vi "PolyTec_Control_Panel.vi"(11 "Settings in":T3={"Name of test"="ScratchPad", "Date"=timestamp(3622387832 s since 1904-01-01), "Location"="Home", "Template"="ScratchPad", "Soundcard"="Babyface Pro (71982712)", "resolution"=32, "Sampling rate"=48000, "Ch1 Gain "=15.0, "Ch2 Gain"=20.0, "Sample time (s)"=0.3, "Pre-trigger (s)"=0.001, "Hammer Threshold"=0.05, "Positions"=1, "Taps/Position"=5, "Set Names"="H", "Freq resolution"=1.0, "Hammer cutoff"=0.03, "Mic cutoff"=0.1, "Double bounce "=0.01, "Hammer Cal"=1.0, "dB Offset"=0.0, "Accel Cal"=1.0, "Vibrometer Cal"=20.0, "Mic Cal"=49.38, "Output"=2, "Voltage Cal"=13.4, "Vibrometer Port"="ASRL27::INSTR", "Range"=4, "High Pass"=2, "Bandwidth"=4, "X Range"=[{"Minimum"=200.0, "Maximum"=10000.0, "Increment"=10.0, "Minor Increment"=100.0, "Start"=200.0}, {"Minimum"=0.0, "Maximum"=0.05, "Increment"=0.025, "Minor Increment"=0.0025, "Start"=0.0}, {"Minimum"=0.0, "Maximum"=0.3, "Increment"=0.1, "Minor Increment"=0.01, "Start"=0.0}, {"Minimum"=200.0, "Maximum"=10000.0, "Increment"=10.0, "Minor Increment"=100.0, "Start"=1000.0}], "Y Range"=[{"Minimum"=-25.0, "Maximum"=0.0, "Increment"=5.0, "Minor Increment"=1.0, "Start"=-25.0}, {"Minimum"=-0.01, "Maximum"=0.1, "Increment"=0.02, "Minor Increment"=0.005, "Start"=0.0}, {"Minimum"=-0.1, "Maximum"=0.1, "Increment"=0.05, "Minor Increment"=0.01, "Start"=-0.1}, {"Minimum"=-61.0, "Maximum"=-21.0, "Increment"=2.0, "Minor Increment"=0.5, "Start"=-60.0}], "dB Spread"=40.0, "Trigger"=0, "Ch_1"=2, "Ch_2"=1, "flip?"=FALSE, "60Hz"=FALSE, "Time offset"=0.0, "Piezo Cal"=1.0, "Default Notes"=""} {"Ch_2" min=1 step=1; "Ch_1" min=1 max=100 step=1; "Trigger" items=["Hammer (force)", "Self-tap", "Spacebar"]; "Bandwidth" items=["1 kHz"=1, "5 kHz"=5, "10 kHz"=10, "25 kHz"=25, "50 kHz"=50, "100 kHz"=100]; "High Pass" items=["Off", "13 Hz", "104 Hz"]; "Range" items=["10 mm/s"=1, "20 mm/s"=2, "50 mm/s"=5, "100 mm/s"=10, "200 mm/s"=20, "500 mm/s"=50, "1 m/s"=100, "2 m/s"=200]; "Output" items=["Accelerometer", "Speed (from acceleration)", "Microphone", "Vibrometer", "Piezo"]; "Voltage Cal" format="%#_13g"; "Ch2 Gain" format="%#_13g"; "Ch1 Gain" format="%#_13g"; "Double bounce" min=0.0; "Mic cutoff" min=0.0 format="%#_4g"; "Hammer cutoff" min=0.0 format="%#_4g"; "Freq resolution" min=0.0; "Pre-trigger (s)" format="%#_13g"; "Date" format="%<%H:%M\n%d/%m/%y>T"; "resolution" items=["16 bit"=16, "24 bit"=24, "32 bit"=32]; "Sampling rate" items=["22050 samp/s"=22050, "44100 samp/s"=44100, "48000 samp/s"=48000]}) -> (1 "Success?":bool, 2 "Updated Settings":T4, 3 "Settings Out":T3={"Name of test"="ScratchPad", "Date"=timestamp(3622387832 s since 1904-01-01), "Location"="Home", "Template"="ScratchPad", "Soundcard"="Babyface Pro (71982712)", "resolution"=32, "Sampling rate"=48000, "Ch1 Gain "=15.0, "Ch2 Gain"=20.0, "Sample time (s)"=0.3, "Pre-trigger (s)"=0.001, "Hammer Threshold"=0.05, "Positions"=1, "Taps/Position"=5, "Set Names"="H", "Freq resolution"=1.0, "Hammer cutoff"=0.03, "Mic cutoff"=0.1, "Double bounce "=0.01, "Hammer Cal"=1.0, "dB Offset"=0.0, "Accel Cal"=1.0, "Vibrometer Cal"=20.0, "Mic Cal"=49.38, "Output"=2, "Voltage Cal"=13.4, "Vibrometer Port"="ASRL27::INSTR", "Range"=4, "High Pass"=2, "Bandwidth"=4, "X Range"=[{"Minimum"=200.0, "Maximum"=10000.0, "Increment"=10.0, "Minor Increment"=100.0, "Start"=200.0}, {"Minimum"=0.0, "Maximum"=0.05, "Increment"=0.025, "Minor Increment"=0.0025, "Start"=0.0}, {"Minimum"=0.0, "Maximum"=0.3, "Increment"=0.1, "Minor Increment"=0.01, "Start"=0.0}, {"Minimum"=200.0, "Maximum"=10000.0, "Increment"=10.0, "Minor Increment"=100.0, "Start"=1000.0}], "Y Range"=[{"Minimum"=-25.0, "Maximum"=0.0, "Increment"=5.0, "Minor Increment"=1.0, "Start"=-25.0}, {"Minimum"=-0.01, "Maximum"=0.1, "Increment"=0.02, "Minor Increment"=0.005, "Start"=0.0}, {"Minimum"=-0.1, "Maximum"=0.1, "Increment"=0.05, "Minor Increment"=0.01, "Start"=-0.1}, {"Minimum"=-61.0, "Maximum"=-21.0, "Increment"=2.0, "Minor Increment"=0.5, "Start"=-60.0}], "dB Spread"=40.0, "Trigger"=0, "Ch_1"=2, "Ch_2"=1, "flip?"=FALSE, "60Hz"=FALSE, "Time offset"=0.0, "Piezo Cal"=1.0, "Default Notes"=""} {"Ch_2" min=1 step=1; "Ch_1" min=1 max=100 step=1; "Trigger" items=["Hammer (force)", "Self-tap", "Spacebar"]; "Bandwidth" items=["1 kHz"=1, "5 kHz"=5, "10 kHz"=10, "25 kHz"=25, "50 kHz"=50, "100 kHz"=100]; "High Pass" items=["Off", "13 Hz", "104 Hz"]; "Range" items=["10 mm/s"=1, "20 mm/s"=2, "50 mm/s"=5, "100 mm/s"=10, "200 mm/s"=20, "500 mm/s"=50, "1 m/s"=100, "2 m/s"=200]; "Output" items=["Accelerometer", "Speed (from acceleration)", "Microphone", "Vibrometer", "Piezo"]; "Voltage Cal" format="%#_13g"; "Ch2 Gain" format="%#_13g"; "Ch1 Gain" format="%#_13g"; "Double bounce" min=0.0; "Mic cutoff" min=0.0 format="%#_4g"; "Hammer cutoff" min=0.0 format="%#_4g"; "Freq resolution" min=0.0; "Pre-trigger (s)" format="%#_13g"; "Date" format="%<%H:%M\n%d/%m/%y>T"; "resolution" items=["16 bit"=16, "24 bit"=24, "32 bit"=32]; "Sampling rate" items=["22050 samp/s"=22050, "44100 samp/s"=44100, "48000 samp/s"=48000]})   [LabVIEW 2022 SP3]
uses:
  PreferencesControl.ctl
  <vilib>/Utility/error.llb/Trim Whitespace One-Sided.vi
panel:
  in  "Serial Connection":bool=TRUE
  in  "Tab Control":enum32{"Serial", "No Serial"}(tab)
  in  "Vibrometer":T1={"Bandwidth"=10, "High Pass"=0, "Range"=50, "Laser"=TRUE, "Beam"=TRUE, "Model"="IVS-500", "Version"="1.0302", "ASE?"=FALSE, "Remote?"=FALSE, "Focus (mm)"={0, 1600, 193}, "Autofocus range (mm)"={0, 1600}, "Baudrate"="9600", "Autofocus"=FALSE} {"Autofocus range (mm)" scale=0.0..1600.0; "Focus (mm)" scale=0.0..1600.0; "Range" items=["10 mm/s"=1, "20 mm/s"=2, "50 mm/s"=5, "100 mm/s"=10, "200 mm/s"=20, "500 mm/s"=50, "1 m/s"=100, "2 m/s"=200]; "High Pass" items=["Off", "13 Hz", "104 Hz"]; "Bandwidth" items=["1 kHz"=1, "5 kHz"=5, "10 kHz"=10, "25 kHz"=25, "50 kHz"=50, "100 kHz"=100]}
  out "Readings":T2={"Temp"=30.2, "Overtemp"=FALSE, "Signal"=8, "Focusing?"=FALSE} {"Signal" scale=0.0..50.0; "Temp" scale=0.0..50.0}
  in  "Port":refnum<visa-resource-name>="No Serial"
  in  "Range (mm/s)":u16
  in  "HP (kHz)":u16
  in  "Bandwidth (kHz)":u16
  out "comm":cluster{"Sent":string, "Received":string}
  in  "Done":bool
  out "FP_max":i32=1600
  out "FP_min":i32
  out "AF min":i32
  # "Vibrometer Settings"
  # "Note:  Some models only go up to 10kHz and 0.5 m/s"
  # "Hz"
  # "dB"
  # "dB"
  # "sec"
  # "sec"
  # "mV/Pa"
  # "mV/m/s2"
  # "mV/mm/s"
  # "V/N"
  # "sec"
  # "sec"
  # "mV/N"
  # "a.u."
  # "a.u."
  # "sec"
  # "Hz"
  # "dB"
  # "dB"
  # "sec"
  # "sec"
  # "mV/Pa"
  # "mV/m/s2"
  # "mV/mm/s"
  # "V/N"
  # "sec"
  # "sec"
  # "mV/N"
  # "a.u."
  # "a.u."
  # "sec"
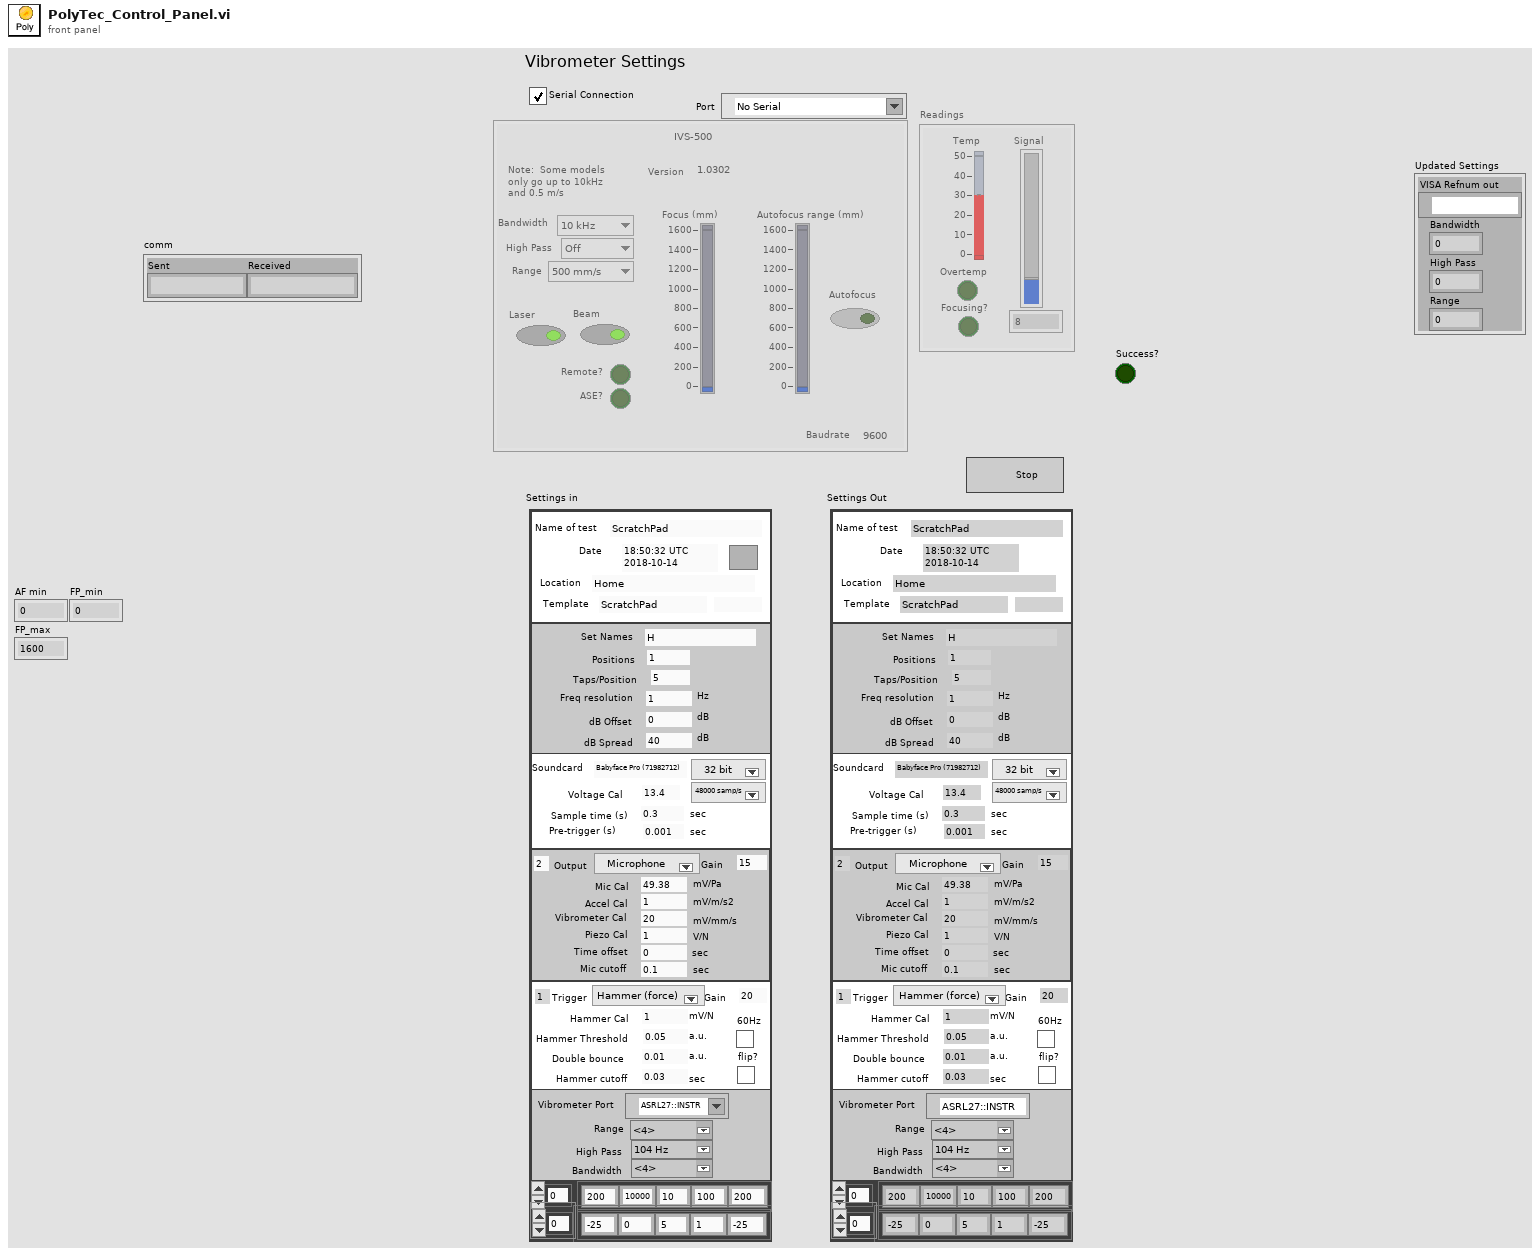
[diagram p1: front panel]
types:
  T1 = cluster{"Bandwidth":u16, "High Pass":u16, "Range":u16, "Laser":bool, "Beam":bool, "Model":string, "Version":string, "ASE?":bool, "Remote?":bool, "Focus (mm)":cluster{u16, u16, u16}, "Autofocus range (mm)":cluster{u16, u16}, "Baudrate":string, "Autofocus":bool}
  T2 = cluster{"Temp":dbl, "Overtemp":bool, "Signal":u8, "Focusing?":bool}
  T3 = typedef "PreferencesControl.ctl" = cluster{"Name of test":string, "Date":timestamp, "Location":string, "Template":string, "Soundcard":string, "resolution":u16, "Sampling rate":u16, "Ch1 Gain ":dbl, "Ch2 Gain":dbl, "Sample time (s)":dbl, "Pre-trigger (s)":dbl, "Hammer Threshold":dbl, "Positions":i16, "Taps/Position":i16, "Set Names":string, "Freq resolution":dbl, "Hammer cutoff":dbl, "Mic cutoff":dbl, "Double bounce ":dbl, "Hammer Cal":dbl, "dB Offset":dbl, "Accel Cal":dbl, "Vibrometer Cal":dbl, "Mic Cal":dbl, "Output":u16, "Voltage Cal":dbl, "Vibrometer Port":refnum<visa-resource-name>, "Range":u16, "High Pass":u16, "Bandwidth":u16, "X Range":cluster{"Minimum":dbl, "Maximum":dbl, "Increment":dbl, "Minor Increment":dbl, "Start":dbl}[], "Y Range":cluster{"Minimum":dbl, "Maximum":dbl, "Increment":dbl, "Minor Increment":dbl, "Start":dbl}[], "dB Spread":dbl, "Trigger":u16, "Ch_1":u8, "Ch_2":u8, "flip?":bool, "60Hz":bool, "Time offset":dbl, "Piezo Cal":dbl, "Default Notes":string}
  T4 = cluster{"VISA Refnum out":refnum<visa-resource-name>, "Bandwidth":u16, "High Pass":u16, "Range":u16}
  T5 = enum8{"Enabled", "Disabled", "Disabled and Grayed Out"}
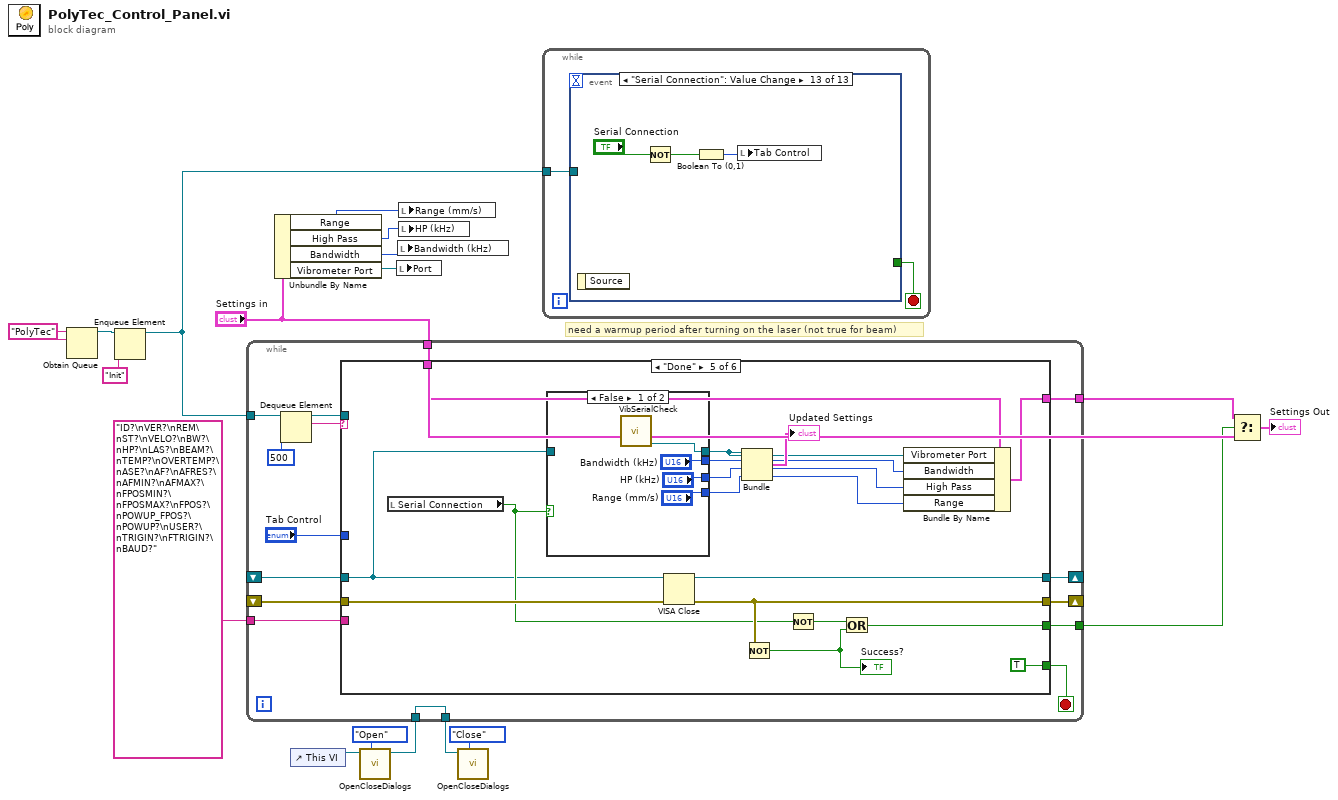
[diagram p0: block diagram]
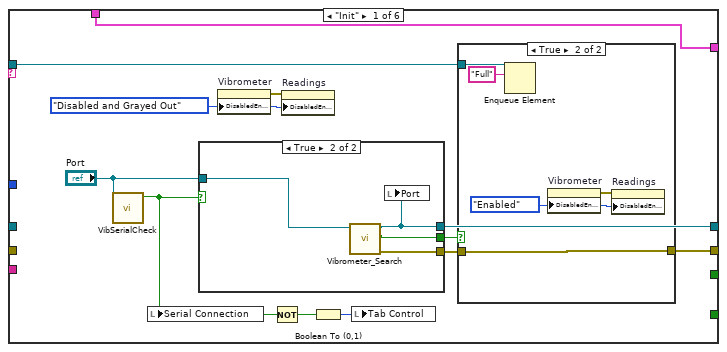
[diagram p2: hidden frame]
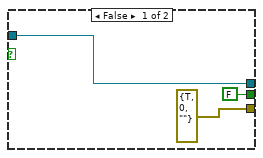
[diagram p3: hidden frame]
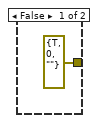
[diagram p4: hidden frame]
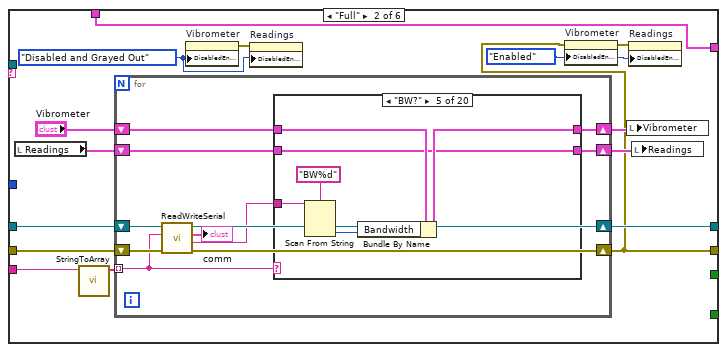
[diagram p5: hidden frame]
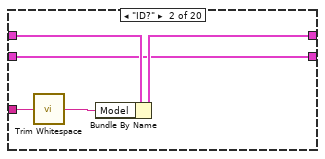
[diagram p7: hidden frame]
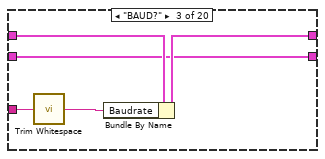
[diagram p8: hidden frame]
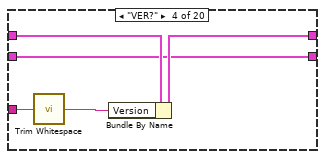
[diagram p9: hidden frame]
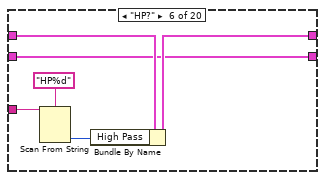
[diagram p10: hidden frame]
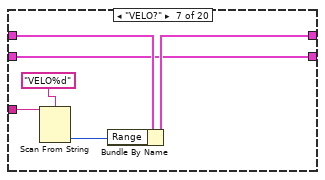
[diagram p11: hidden frame]
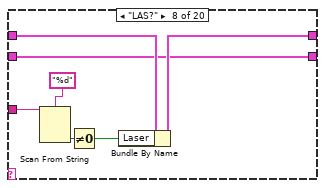
[diagram p12: hidden frame]
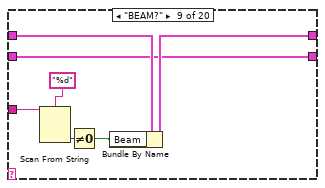
[diagram p13: hidden frame]
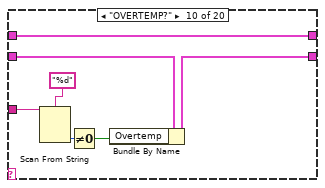
[diagram p14: hidden frame]
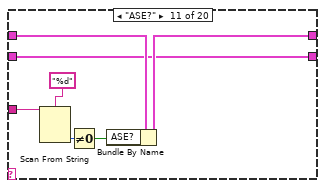
[diagram p15: hidden frame]
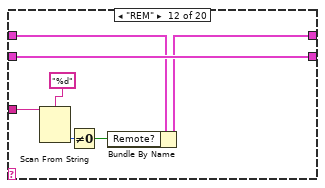
[diagram p16: hidden frame]
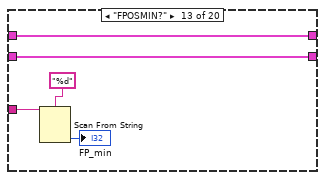
[diagram p17: hidden frame]
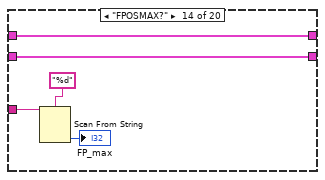
[diagram p18: hidden frame]
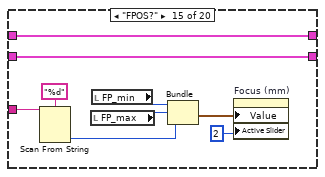
[diagram p19: hidden frame]
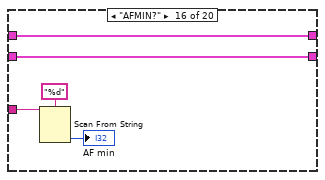
[diagram p20: hidden frame]
diagram:
  w17 = "PolyTec" ("name (unnamed)")
  # "need a warmup period after turning on the laser (not true for beam)"
  n1 = Obtain Queue(name (unnamed)=w17, element data type=w17) -> (queue out=w15:refnum<queue>)  [unwired: 3 in, 2 out]
  n2 = Enqueue Element(queue=w15, element="Init") -> (queue out=w18:refnum<queue>)  [unwired: 2 in, 2 out]
  n3 = Unbundle By Name("Settings in") -> ("Range"=w8:u16, "High Pass"=w7:u16, "Bandwidth"=w6:u16, "Vibrometer Port"=w10:refnum<visa-resource-name>)
  n4 = control-ref of="This VI"() -> (w4:refnum<vi>)
  n5 = call "OpenCloseDialogs.vi"("Task"=enum16{"Open", "Close"}."Open", "VI in"=w4) -> ("VI out"=w1:refnum<vi>)  [unwired: 8 in, 1 out]
  n6 = while {
    tunnel: w18 -> [w33]
    shift-right: [w31] -> _
    shift-left: _ -> [w30]
    shift-right: [w29] -> _
    shift-left: _ -> [w28]
    tunnel: "ID?\nVER?\nREM\nST?\nVELO?\nBW?\nHP?\nLAS?\nBEAM?\nTEMP?\nOVERTEMP?\nASE?\nAF?\nAFRES?\nAFMIN?\nAFMAX?\nFPOSMIN?\nFPOSMAX?\nFPOS?\nPOWUP_FPOS?\nPOWUP?\nUSER?\nTRIGIN?\nFTRIGIN?\nBAUD?" ("write buffer") -> [w24]
    tunnel: "Settings in" -> [w23]
    tunnel: [w22] -> w13
    tunnel: [w20] -> w9
    tunnel: [w19] -> w2
    tunnel: w1 -> [w19]
    stop <- w26 stop-if-true
    n7 = Dequeue Element(queue=w33, timeout in ms (-1)=500) -> (queue out=w25:refnum<queue>, element=w32:string)  [unwired: 1 in, 2 out]
    n8 = case shown="\"Done\"" w32 {
      selector: w32 -> [_ _ w208 _ _ _]
      tunnel: [w41 w70 w211 w225 w235 w260] -> w31
      tunnel: w30 -> [_ w69 w212 w227 w235 w260]
      tunnel: [w43 w61 w209 w224 w238 w262] -> w29
      tunnel: w28 -> [_ w68 w210 w226 w239 w262]
      tunnel: [_ _ _ _ TRUE TRUE] -> w26
      tunnel: w25 -> [w42 _ _ _ _ _]
      tunnel: w24 -> [_ w60 _ _ _ _]
      tunnel: w23 -> [w38 w59 w207 w223 w244 w259]
      tunnel: [w38 w59 w207 w223 w243 w259] -> w22
      tunnel: "Tab Control" -> [_ _ w206 w222 _ _]
      tunnel: [_ _ _ _ w241 _] -> w20
      frame "Init" {
        w44 = T5."Disabled and Grayed Out" ("Disabled")
        n9 = call "VibSerialCheck.vi"("VISA Refnum in"="Port") -> ("Serial?"=w34:bool)  [unwired: 9 in, 1 out]
        n10 = local write "Serial Connection"(w34) -> ()
        n11 = case shown="True" w34 {
          tunnel: [w48 w52] -> w41
          tunnel: [FALSE ("Success?") w51] -> w40
          tunnel: [errorcluster {"status"=TRUE, "code"=0, "source"=""} ("error out") w50] -> w39
          tunnel: "Port" -> [w48 w49]
          frame False {
          }
          frame True {
            n12 = call "Vibrometer_Search.vi"("VISA Refnum in"=w49) -> ("error out"=w50:errorcluster, "Success?"=w51:bool, "VISA Refnum out"=w52:refnum<visa-resource-name>)  [unwired: 8 in]
            n13 = local write "Port"(w52) -> ()
          }
        }
        n14 = property on="Vibrometer" class="Clust (strict)"("DisabledEnum"=w44) -> (error out=w45:errorcluster)  [unwired: 2 in, 1 out]
        n15 = Not(x=w34) -> (.not. x?=w36:bool)
        n16 = property on="Readings" class="Clust (strict)"(error in=w45, "DisabledEnum"=w44) -> ()  [unwired: 1 in, 2 out]
        n17 = Boolean To (0,1)(Boolean=w36) -> (0, 1=w37:i16)
        n18 = local write "Tab Control"(w37) -> ()
        n19 = case shown="True" w40 {
          tunnel: [errorcluster {"status"=TRUE, "code"=0, "source"=""} ("error out") w54] -> w43
          tunnel: w42 -> [_ w55]
          tunnel: w39 -> [_ w54]
          frame False {
          }
          frame True {
            w57 = T5."Enabled" ("Disabled")
            n20 = Enqueue Element(queue=w55, element="Full") -> ()  [unwired: 2 in, 3 out]
            n21 = property on="Vibrometer" class="Clust (strict)"("DisabledEnum"=w57) -> (error out=w58:errorcluster)  [unwired: 2 in, 1 out]
            n22 = property on="Readings" class="Clust (strict)"(error in=w58, "DisabledEnum"=w57) -> ()  [unwired: 1 in, 2 out]
          }
        }
      }
      frame "Full" {
        w62 = T5."Enabled" ("Disabled")
        w64 = T5."Disabled and Grayed Out" ("Disabled")
        n23 = local read "Readings"() -> (w71:T2)
        n24 = call "StringToArray.vi"("write buffer"=w60) -> ("Array"=w73:string[])  [unwired: 10 in]
        n25 = for {
          tunnel: w73 -> [w80] mode=indexing
          shift-right: [w84] -> w61
          shift-left: w68 -> [w82]
          shift-right: [w83] -> w70
          shift-left: w69 -> [w81]
          shift-right: [w77] -> w66
          shift-left: "Vibrometer" -> [w78]
          shift-right: [w75] -> w67
          shift-left: w71 -> [w76]
          n26 = call "ReadWriteSerial.vi"("error in (no error)"=w82, "cmd"=w80, "VISA Refnum in"=w81) -> ("error out"=w84:errorcluster, "Reply"=w79:string, "comm"=→"comm":cluster{"Sent":string, "Received":string}, "VISA Refnum out"=w83:refnum<visa-resource-name>)  [unwired: 5 in]
          n27 = case shown="\"BW?\"" w80 {
            tunnel: w79 -> [_ w91 w96 w101 w107 w113 w119 w126 w133 w140 w147 w154 w159 w164 w173 w178 w186 w193 w199 w205]
            tunnel: w78 -> [w86 w90 w95 w100 w104 w110 w117 w122 w129 w137 w143 w149 w156 w161 w166 w175 w180 w189 w197 w203]
            tunnel: [w86 w89 w94 w99 w103 w109 w115 w121 w128 w137 w142 w148 w156 w161 w166 w175 w180 w189 w197 w203] -> w77
            tunnel: w76 -> [w85 w87 w92 w97 w102 w108 w114 w120 w127 w136 w141 w151 w155 w160 w165 w174 w179 w188 w196 w201]
            tunnel: [w85 w87 w92 w97 w102 w108 w114 w120 w127 w135 w141 w151 w155 w160 w165 w174 w179 w187 w194 w200] -> w75
            frame Default {
            }
            frame "ID?" {
              n28 = call <vilib>:"Trim Whitespace.vi"("string"=w91) -> ("trimmed string"=w88:string)  [unwired: 1 in]
              n29 = Bundle By Name(cluster=w90, "Model"=w88) -> (w89:T1)
            }
            frame "BAUD?" {
              n30 = call <vilib>:"Trim Whitespace.vi"("string"=w96) -> ("trimmed string"=w93:string)  [unwired: 1 in]
              n31 = Bundle By Name(cluster=w95, "Baudrate"=w93) -> (w94:T1)
            }
            frame "VER?" {
              n32 = call <vilib>:"Trim Whitespace.vi"("string"=w101) -> ("trimmed string"=w98:string)  [unwired: 1 in]
              n33 = Bundle By Name(cluster=w100, "Version"=w98) -> (w99:T1)
            }
            frame "BW?" {
              n34 = Scan From String(format string="BW%d", input string=w107) -> (output 1=w105:i32)  [unwired: 3 in, 3 out]
              n35 = Bundle By Name(cluster=w104, "Bandwidth"=w105) -> (w103:T1)
            }
            frame "HP?" {
              n36 = Scan From String(format string="HP%d", input string=w113) -> (output 1=w111:i32)  [unwired: 3 in, 3 out]
              n37 = Bundle By Name(cluster=w110, "High Pass"=w111) -> (w109:T1)
            }
            frame "VELO?" {
              n38 = Scan From String(format string="VELO%d", input string=w119) -> (output 1=w116:i32)  [unwired: 3 in, 3 out]
              n39 = Bundle By Name(cluster=w117, "Range"=w116) -> (w115:T1)
            }
            frame "LAS?" {
              n40 = Scan From String(format string="%d", input string=w126) -> (output 1=w124:i32)  [unwired: 3 in, 3 out]
              n41 = Not Equal To 0?(x=w124) -> (x != 0?=w123:bool)
              n42 = Bundle By Name(cluster=w122, "Laser"=w123) -> (w121:T1)
            }
            frame "BEAM?" {
              n43 = Scan From String(format string="%d", input string=w133) -> (output 1=w131:i32)  [unwired: 3 in, 3 out]
              n44 = Not Equal To 0?(x=w131) -> (x != 0?=w130:bool)
              n45 = Bundle By Name(cluster=w129, "Beam"=w130) -> (w128:T1)
            }
            frame "OVERTEMP?" {
              n46 = Scan From String(format string="%d", input string=w140) -> (output 1=w138:i32)  [unwired: 3 in, 3 out]
              n47 = Not Equal To 0?(x=w138) -> (x != 0?=w134:bool)
              n48 = Bundle By Name(cluster=w136, "Overtemp"=w134) -> (w135:T2)
            }
            frame "ASE?" {
              n49 = Scan From String(format string="%d", input string=w147) -> (output 1=w145:i32)  [unwired: 3 in, 3 out]
              n50 = Not Equal To 0?(x=w145) -> (x != 0?=w144:bool)
              n51 = Bundle By Name(cluster=w143, "ASE?"=w144) -> (w142:T1)
            }
            frame "REM" {
              n52 = Scan From String(format string="%d", input string=w154) -> (output 1=w152:i32)  [unwired: 3 in, 3 out]
              n53 = Not Equal To 0?(x=w152) -> (x != 0?=w150:bool)
              n54 = Bundle By Name(cluster=w149, "Remote?"=w150) -> (w148:T1)
            }
            frame "FPOSMIN?" {
              n55 = Scan From String(format string="%d", input string=w159) -> (output 1=→"FP_min":i32)  [unwired: 3 in, 3 out]
            }
            frame "FPOSMAX?" {
              n56 = Scan From String(format string="%d", input string=w164) -> (output 1=→"FP_max":i32)  [unwired: 3 in, 3 out]
            }
            frame "FPOS?" {
              n57 = Scan From String(format string="%d", input string=w173) -> (output 1=w169:i32)  [unwired: 3 in, 3 out]
              n58 = local read "FP_max"() -> (w170:i32)
              n59 = local read "FP_min"() -> (w171:i32)
              n60 = Bundle("FP_min"=w171, "FP_max"=w170, w169) -> (w168:cluster{"FP_min":i32, "FP_max":i32, i32})  [unwired: 1 in]
              n61 = property on="Focus (mm)" class="Slide (strict)"("Value"=w168, "Active Slider"=2) -> ()  [unwired: 2 in, 2 out]
            }
            frame "AFMIN?" {
              n62 = Scan From String(format string="%d", input string=w178) -> (output 1=→"AF min":i32)  [unwired: 3 in, 3 out]
            }
            frame "AFMAX?" {
              n63 = Scan From String(format string="%d", input string=w186) -> (output 1=w182:i32)  [unwired: 3 in, 3 out]
              n64 = local read "AF min"() -> (w183:i32)
              n65 = Bundle("AF min"=w183, w182) -> (w181:cluster{"AF min":i32, i32})  [unwired: 1 in]
              n66 = property on="Autofocus range (mm)" class="Slide (strict)"("Active Slider"=1, "Value"=w181) -> ()  [unwired: 2 in, 2 out]
            }
            frame "AF?" {
              n67 = Scan From String(format string="%d", input string=w193) -> (output 1=w191:i32)  [unwired: 3 in, 3 out]
              n68 = Not Equal To 0?(x=w191) -> (x != 0?=w190:bool)
              n69 = Bundle By Name(cluster=w188, "Focusing?"=w190) -> (w187:T2)
            }
            frame "TEMP?" {
              n70 = Scan From String(format string="%f", input string=w199) -> (output 1=w195:dbl)  [unwired: 3 in, 3 out]
              n71 = Bundle By Name(cluster=w196, "Temp"=w195) -> (w194:T2)
            }
            frame "ST?" {
              n72 = Scan From String(format string="%d", input string=w205) -> (output 1=w202:i32)  [unwired: 3 in, 3 out]
              n73 = Bundle By Name(cluster=w201, "Signal"=w202) -> (w200:T2)
            }
          }
        }
        n74 = property on="Vibrometer" class="Clust (strict)"("DisabledEnum"=w64) -> (error out=w65:errorcluster)  [unwired: 2 in, 1 out]
        n75 = property on="Readings" class="Clust (strict)"(error in=w65, "DisabledEnum"=w64) -> ()  [unwired: 1 in, 2 out]
        n76 = property on="Vibrometer" class="Clust (strict)"(error in=w61, "DisabledEnum"=w62) -> (error out=w63:errorcluster)  [unwired: 1 in, 1 out]
        n77 = local write "Vibrometer"(w66) -> ()
        n78 = property on="Readings" class="Clust (strict)"(error in=w63, "DisabledEnum"=w62) -> ()  [unwired: 1 in, 2 out]
        n79 = local write "Readings"(w67) -> ()
      }
      frame Default {
        n80 = case shown="\"Serial\", Default" w206 {
          tunnel: w212 -> [w218 w221]
          tunnel: [w217 w221] -> w211
          tunnel: w210 -> [w216 w220]
          tunnel: [w215 w220] -> w209
          tunnel: w208 -> [w214 _]
          frame "Serial", Default {
            n81 = call "ReadWriteSerial.vi"("error in (no error)"=w216, "cmd"=w214, "VISA Refnum in"=w218) -> ("error out"=w215:errorcluster, "comm"=w213:cluster{"Sent":string, "Received":string}, "VISA Refnum out"=w217:refnum<visa-resource-name>)  [unwired: 5 in, 1 out]
            n82 = local write "comm"(w213) -> ()
            n83 = flat-sequence {
              tunnel: w213 -> [_]
              frame #0 {
                n84 = property on="Autofocus" class="Bool (strict)"("Value"=FALSE) -> ()  [unwired: 2 in, 2 out]
              }
            }
          }
          frame "No Serial" {
          }
        }
      }
      frame "" {
        n85 = case shown="\"Serial\", Default" w222 {
          tunnel: w227 -> [w231 w234]
          tunnel: w226 -> [w230 w233]
          tunnel: [w229 w234] -> w225
          tunnel: [w228 w233] -> w224
          frame "Serial", Default {
            n86 = call "Updates.vi"("error in (no error)"=w230, "VISA Refnum in"=w231) -> ("error out"=w228:errorcluster, "Readings out"=→"Readings":T2, "VISA Refnum out"=w229:refnum<visa-resource-name>)  [unwired: 7 in]
          }
          frame "No Serial" {
          }
        }
      }
      frame "Done" {
        n87 = local read "Serial Connection"() -> (w237:bool)
        n88 = case shown="False" w237 {
          tunnel: ["Bandwidth (kHz)" w257] -> w247
          tunnel: ["HP (kHz)" w256] -> w246
          tunnel: ["Range (mm/s)" w255] -> w245
          tunnel: [w250 w254] -> w236
          tunnel: w235 -> [_ w254]
          frame False {
            n89 = call "VibSerialCheck.vi"() -> ("NoSerial"=w250:refnum<visa-resource-name>)  [unwired: 10 in, 1 out]
          }
          frame True {
            n90 = local read "Vibrometer"() -> (w258:T1)
            n91 = Unbundle By Name(w258) -> ("Bandwidth"=w257:u16, "High Pass"=w256:u16, "Range"=w255:u16)
          }
        }
        n92 = VISA Close(VISA resource name=w235, error in (no error)=w239) -> (error out=w238:errorcluster)
        n93 = Bundle("VISA Refnum out"=w236, "Bandwidth"=w247, "High Pass"=w246, "Range"=w245) -> (→"Updated Settings":T4)  [unwired: 1 in]
        n94 = Not(x=w238) -> (.not. x?=w242:bool)
        "Success?" <- w242
        n95 = Not(x=w237) -> (.not. x?=w240:bool)
        n96 = Or(x=w240, y=w242) -> (x .or. y?=w241:bool)
        n97 = Bundle By Name(cluster=w244, "Vibrometer Port"=w236, "Bandwidth"=w247, "High Pass"=w246, "Range"=w245) -> (w243:T3)
      }
      frame "Revert" {
      }
    }
  }
  n98 = local write "Port"(w10) -> ()
  n99 = local write "Bandwidth (kHz)"(w6) -> ()
  n100 = local write "Range (mm/s)"(w8) -> ()
  n101 = local write "HP (kHz)"(w7) -> ()
  n102 = call "OpenCloseDialogs.vi"("Task"=enum16{"Open", "Close"}."Close", "VI in"=w2) -> ()  [unwired: 8 in, 2 out]
  n103 = while {
    tunnel: w18 -> [w263]
    stop <- w264 stop-if-true
    n104 = event shown="[12] \"Serial Connection\": Value Change" {
      selector: _ -> [_ _ _ _ _ _ _ _ _ _ _ _ _]
      dyn-events: _ -> [_ _ _ _ _ _ _ _ _ _ _ _ _]
      timeout: _ -> [_ _ _ _ _ _ _ _ _ _ _ _ _]
      tunnel: [_ "Done" w268 _ _ _ _ _ _ _ _ _ _] -> w264
      tunnel: w263 -> [_ w266 w270 w271 w273 w278 w286 w293 w299 w305 w309 w323 _]
      event Timeout {
        n105 = event-data() -> ()  [unwired: 1 in, 1 out]
      }
      event "Done": Value Change {
        n106 = event-data() -> ()  [unwired: 1 in, 1 out]
        n107 = Enqueue Element(queue=w266, element="Done") -> ()  [unwired: 2 in, 3 out]
      }
      event Panel Close? {
        w268 = TRUE ("Discard?")
        n108 = event-data() -> ()  [unwired: 1 in, 1 out]
        n109 = Enqueue Element(queue=w270, element="Revert") -> ()  [unwired: 2 in, 3 out]
        n110 = event-data("Discard?"=w268) -> ()  [unwired: 1 in, 1 out]
      }
      event "Port": Value Change {
        n111 = event-data() -> ()  [unwired: 1 in, 1 out]
        n112 = Enqueue Element(queue=w271, element="Init") -> ()  [unwired: 2 in, 3 out]
      }
      event "Vibrometer.Laser": Value Change {
        n113 = event-data() -> ("NewVal"=w277:bool)  [unwired: 1 in]
        n114 = Boolean To (0,1)(Boolean=w277) -> (0, 1=w276:i16)
        n115 = Format Into String(format string="LAS%d", w276) -> (resulting string=w274:string)  [unwired: 2 in, 1 out]
        n116 = Enqueue Element(queue=w273, element=w274) -> ()  [unwired: 2 in, 3 out]
      }
      event "Vibrometer.Beam": Value Change {
        n117 = event-data() -> ("NewVal"=w282:bool)  [unwired: 1 in]
        n118 = Boolean To (0,1)(Boolean=w282) -> (0, 1=w281:i16)
        n119 = Format Into String(format string="BEAM%d", w281) -> (resulting string=w279:string)  [unwired: 2 in, 1 out]
        n120 = Enqueue Element(queue=w278, element=w279) -> ()  [unwired: 2 in, 3 out]
      }
      event "Vibrometer.Autofocus": Value Change {
        n121 = event-data() -> ("NewVal"=w289:bool)  [unwired: 1 in]
        n122 = Boolean To (0,1)(Boolean=w289) -> (0, 1=w288:i16)
        n123 = Format Into String(format string="AF%d", w288) -> (resulting string=w285:string)  [unwired: 2 in, 1 out]
        n124 = Enqueue Element(queue=w286, element=w285) -> (queue out=w284:refnum<queue>)  [unwired: 2 in, 2 out]
        n125 = Enqueue Element(queue=w284, element="Full" ("format string")) -> ()  [unwired: 2 in, 3 out]
      }
      event "Vibrometer.Bandwidth": Value Change {
        n126 = event-data() -> ("NewVal"=w294:u16)  [unwired: 1 in]
        n127 = Format Into String(format string="BW%d", w294) -> (resulting string=w292:string)  [unwired: 2 in, 1 out]
        n128 = Enqueue Element(queue=w293, element=w292) -> (queue out=w291:refnum<queue>)  [unwired: 2 in, 2 out]
        n129 = Enqueue Element(queue=w291, element="Full" ("format string")) -> ()  [unwired: 2 in, 3 out]
      }
      event "Vibrometer.High Pass": Value Change {
        n130 = event-data() -> ("NewVal"=w300:u16)  [unwired: 1 in]
        n131 = Format Into String(format string="HP%d", w300) -> (resulting string=w298:string)  [unwired: 2 in, 1 out]
        n132 = Enqueue Element(queue=w299, element=w298) -> (queue out=w296:refnum<queue>)  [unwired: 2 in, 2 out]
        n133 = Enqueue Element(queue=w296, element="Full" ("format string")) -> ()  [unwired: 2 in, 3 out]
      }
      event "Vibrometer.Range": Value Change {
        n134 = event-data() -> ("NewVal"=w306:u16)  [unwired: 1 in]
        n135 = Format Into String(format string="VELO%d", w306) -> (resulting string=w304:string)  [unwired: 2 in, 1 out]
        n136 = Enqueue Element(queue=w305, element=w304) -> (queue out=w302:refnum<queue>)  [unwired: 2 in, 2 out]
        n137 = Enqueue Element(queue=w302, element="Full" ("format string")) -> ()  [unwired: 2 in, 3 out]
      }
      event "Vibrometer.Focus (mm)": Mouse Up {
        n138 = event-data() -> ()  [unwired: 1 in, 1 out]
        n139 = property on="Focus (mm)" class="Slide (strict)"() -> ("Value"=w308:cluster{u16, u16, u16})  [unwired: 2 in, 2 out]
        n140 = Unbundle(w308) -> (w314:u16, w313:u16, w312:u16)
        n141 = Format Into String(format string="FPOSMIN_%d\nFPOSMAX_%d\nFPOS_%d", w314, w313, w312) -> (resulting string=w311:string)  [unwired: 2 in, 1 out]
        n142 = call "StringToArray.vi"("write buffer"=w311) -> ("Array"=w310:string[])  [unwired: 10 in]
        n143 = for {
          tunnel: w310 -> [w317] mode=indexing
          tunnel: w309 -> [w316]
          n144 = Enqueue Element(queue=w316, element=w317) -> ()  [unwired: 2 in, 3 out]
        }
      }
      event "Vibrometer.Autofocus range (mm)": Mouse Up {
        n145 = event-data() -> ()  [unwired: 1 in, 1 out]
        n146 = property on="Autofocus range (mm)" class="Slide (strict)"() -> ("Value"=w320:cluster{u16, u16})  [unwired: 2 in, 2 out]
        n147 = Unbundle(w320) -> (w319:u16, w318:u16)
        n148 = Format Into String(format string="AFMIN%d\nAFMAX%d", w319, w318) -> (resulting string=w325:string)  [unwired: 2 in, 1 out]
        n149 = call "StringToArray.vi"("write buffer"=w325) -> ("Array"=w324:string[])  [unwired: 10 in]
        n150 = for {
          tunnel: w324 -> [w328] mode=indexing
          tunnel: w323 -> [w329]
          tunnel: [w327] -> w321
          n151 = Enqueue Element(queue=w329, element=w328) -> (queue out=w327:refnum<queue>)  [unwired: 2 in, 2 out]
        }
        n152 = Enqueue Element(queue=w321, element="Full" ("format string")) -> ()  [unwired: 2 in, 3 out]
      }
      event "Serial Connection": Value Change {
        n153 = event-data() -> ()  [unwired: 1 in, 1 out]
        n154 = Not(x="Serial Connection") -> (.not. x?=w330:bool)
        n155 = Boolean To (0,1)(Boolean=w330) -> (0, 1=w331:i16)
        n156 = local write "Tab Control"(w331) -> ()
      }
    }
  }
  n157 = Select(t=w13, s=w9, f="Settings in") -> (s? t:f=→"Settings Out":T3)
